vi "PlayfieldUpdate.vi"(8 "TetroInfo New":T1, 9 "TetroInfo Old":T1, 11 "Playfield Input":bool[][](array[boolean])) -> (3 "Playfield Output":bool[][](array[boolean]))   [LabVIEW 2026]
doc: "This VI updates the playfield according to the new calculated coordinates of the falling tetromino."
uses:
  02_StateMachine/GameTetrominoInformationTypeDef.ctl
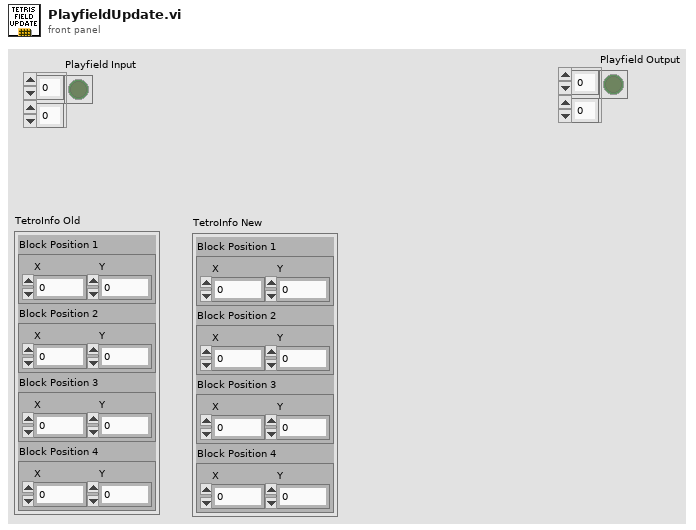
[diagram p1: front panel]
types:
  T1 = typedef "GameTetrominoInformationTypeDef.ctl" = cluster{"Block Position 1":cluster{"X":i32, "Y":i32}, "Block Position 2":cluster{"X":i32, "Y":i32}, "Block Position 3":cluster{"X":i32, "Y":i32}, "Block Position 4":cluster{"X":i32, "Y":i32}}
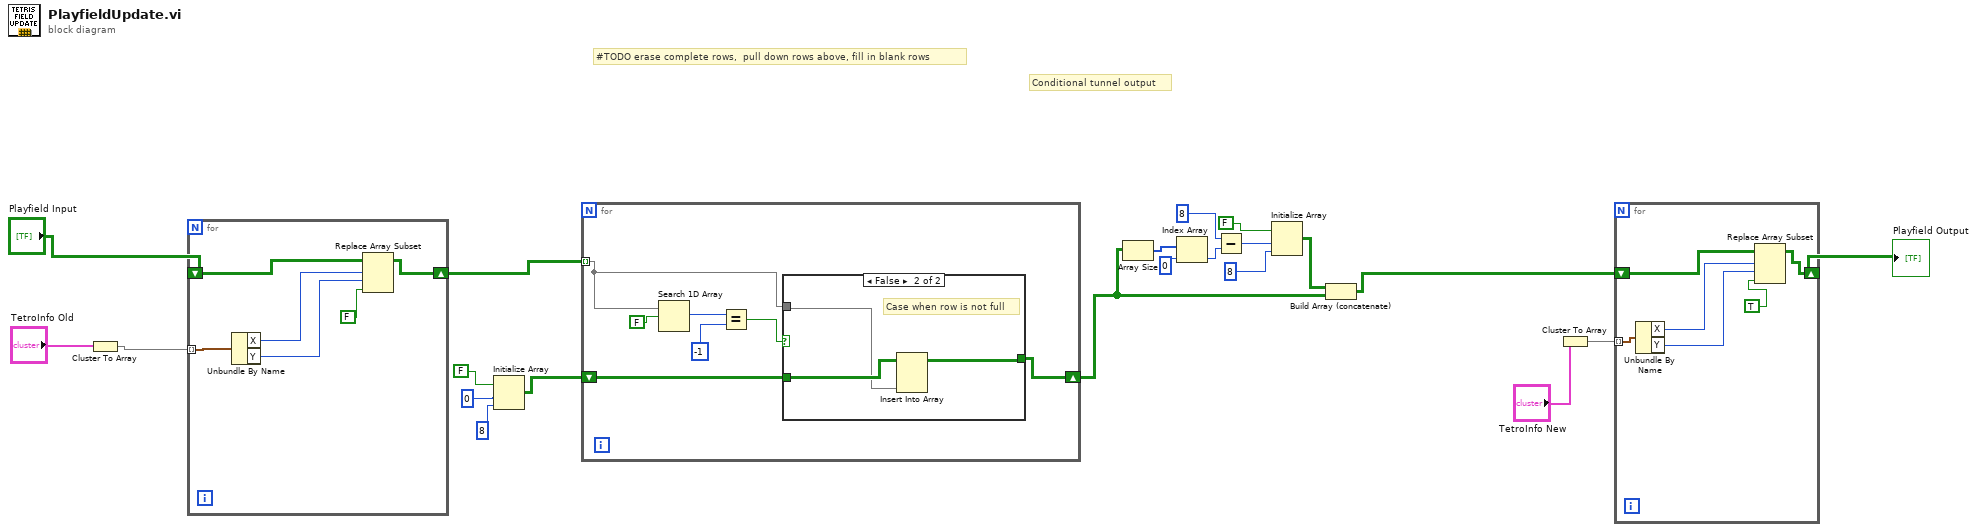
[diagram p0: block diagram]
diagram:
  # "Conditional tunnel output"
  # "#TODO erase complete rows,  pull down rows above, fill in blank rows"
  n1 = Cluster To Array(cluster="TetroInfo Old") -> (array=w20:cluster{"X":i32, "Y":i32}[])
  n2 = for {
    tunnel: w20 -> [w27] mode=indexing
    shift-right: [w23] -> w14
    shift-left: "Playfield Input" -> [w26]
    n3 = Unbundle By Name(w27) -> ("X"=w25:i32, "Y"=w24:i32)
    n4 = Replace Array Subset(array=w26, new element=FALSE ("new element/subarray"), index (row)=w25, index (col)=w24) -> (w23:bool[][])
  }
  n5 = Initialize Array(FALSE, 0 ("dimension size"), 8 ("dimension size")) -> (w13:bool[][])
  n6 = for {
    tunnel: w14 -> [w29] mode=indexing
    shift-right: [w28] -> w6
    shift-left: w13 -> [w34]
    n7 = Search 1D Array(1D array=w29, element=FALSE) -> (index of element=w32:i32)  [unwired: 1 in]
    n8 = Equal?(x=w32, y=-1) -> (x = y?=w30:bool)
    n9 = case shown="False" w30 {
      tunnel: [w35 w38] -> w28
      tunnel: w34 -> [w35 w37]
      tunnel: w29 -> [_ w36]
      frame True {
        # "Case when row is full"
      }
      frame False {
        # "Case when row is not full"
        n10 = Insert Into Array(array=w37, new element=w36) -> (w38:bool[][])  [unwired: 2 in]
      }
    }
  }
  n11 = Array Size(array=w6) -> (size(s)=w5:i32[])
  n12 = Index Array(array=w5, index=0) -> (element=w2:i32)
  n13 = Subtract(x=8, y=w2) -> (x-y=w3:i32)
  n14 = Initialize Array(FALSE, w3, 8 ("dimension size")) -> (w9:bool[][])
  n15 = Build Array (concatenate)(w9, w6) -> (w15:bool[][])
  n16 = Cluster To Array(cluster="TetroInfo New") -> (array=w17:cluster{"X":i32, "Y":i32}[])
  n17 = for {
    tunnel: w17 -> [w41] mode=indexing
    shift-right: [w39] -> w16
    shift-left: w15 -> [w40]
    n18 = Unbundle By Name(w41) -> ("X"=w44:i32, "Y"=w43:i32)
    n19 = Replace Array Subset(array=w40, new element=TRUE ("new element/subarray"), index (row)=w44, index (col)=w43) -> (w39:bool[][])
  }
  "Playfield Output" <- w16
